vi "Analyze.vi"(11 "Queues":T1) -> ()   [LabVIEW 2014]
uses:
  CMD UI enum.ctl
  CMD Report enum.ctl
  CMD DA enum.ctl
  CMD DAQ enum.ctl
  CMD LOG enum.ctl
  patiant and daq params.ctl
  set-get-size.ctl
  set_get.ctl
  <vilib>/Analysis/baseanly.llb/Mean (DBL).vi
  <vilib>/Analysis/NI_AALBase.lvlib
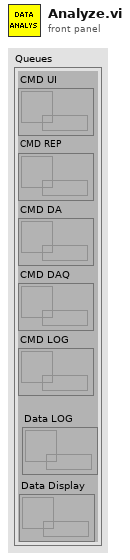
[diagram p1: front panel]
types:
  T1 = cluster{"CMD UI":refnum<queue>, "CMD REP":refnum<queue>, "CMD DA":refnum<queue>, "CMD DAQ":refnum<queue>, "CMD LOG":refnum<queue>, "Data LOG":refnum<queue>, "Data Display":refnum<queue>}
  T2 = typedef "CMD DA enum.ctl" = enum16{"Wait", "Analyze", "Meta Analyze", "Exit"}
  T3 = typedef "patiant and daq params.ctl" = cluster{"DAQ Parameters":cluster{"Sampling rate":dbl, "Max_volt":dbl, "Min_volt":dbl, "DAQmx Physical Channels \nHR,SC":tag, "Resting State":bool, "Analyze every (s)":dbl}, "Patient Info \n(Updates automatically when reading from file)":cluster{"Patient Name":string, "Patient ID":string, "Patient Age":dbl, "Gender":string}, "Raw Data Read Path":path, "Avg HR ":dbl, "Avg SC  ":dbl}
  T4 = typedef "set-get-size.ctl" = enum16{"set", "get", "size"}
  T5 = typedef "set_get.ctl" = enum16{"Set", "Get"}
  T6 = typedef "CMD UI enum.ctl" = enum16{"Init all", "Update Patient Info", "Update Analyzed", "Create Report", "Analyze Data", "Start DAQ", "Start Read", "LOG Data", "Stop LOG Data", "Stop DAQ", "Stop Read", "EXIT"}
  T7 = cluster{bool, bool, bool, "mean":dbl, "mean":dbl}
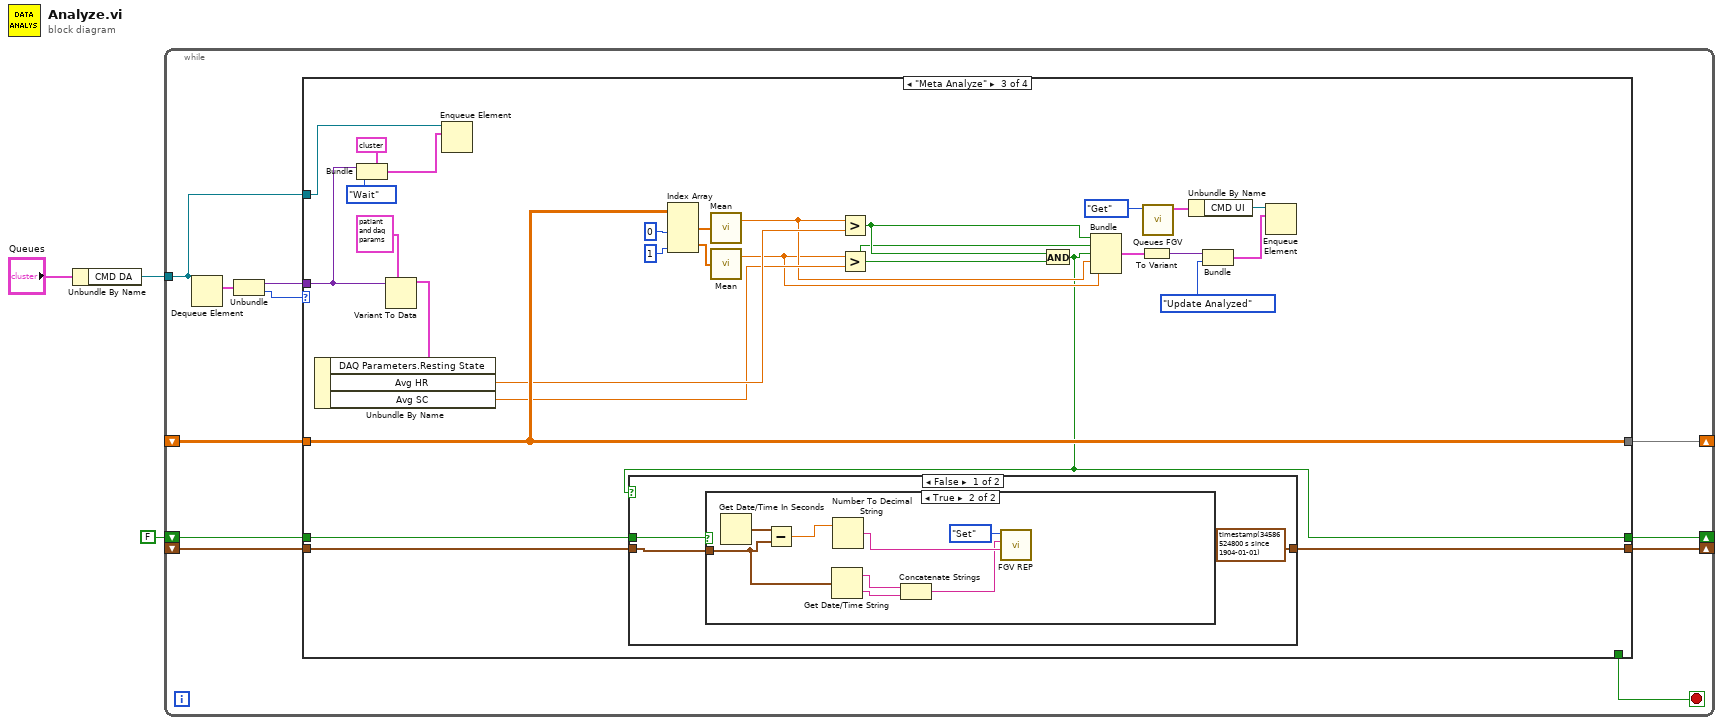
[diagram p0: block diagram]
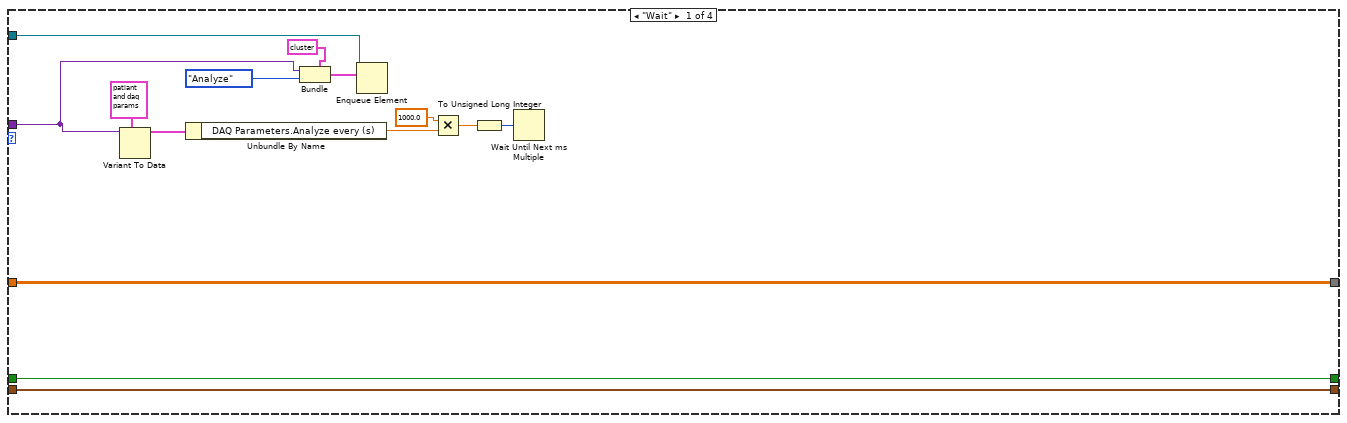
[diagram p2: hidden frame]
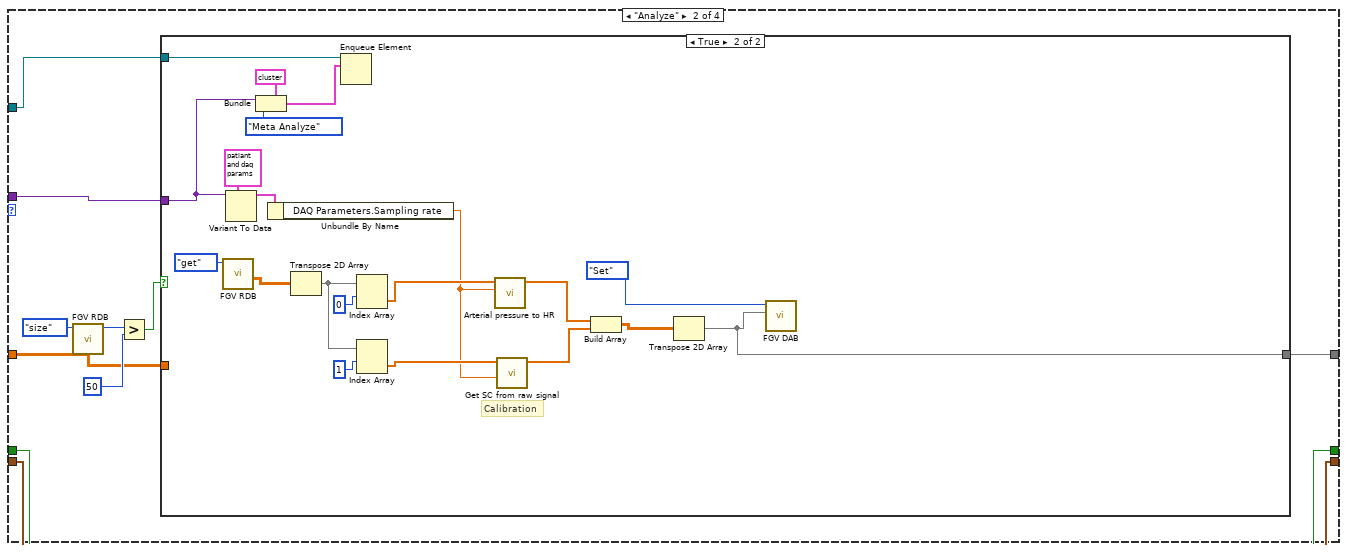
[diagram p3: hidden frame]
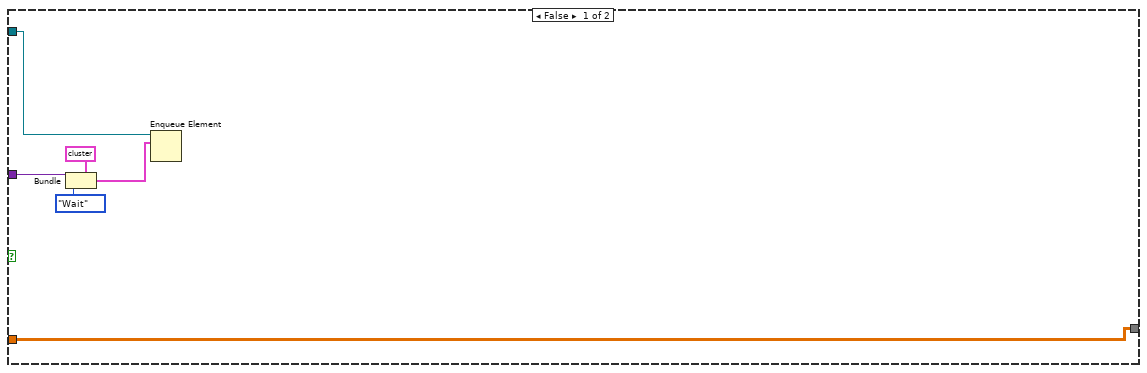
[diagram p4: hidden frame]
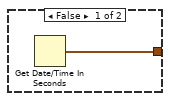
[diagram p7: hidden frame]
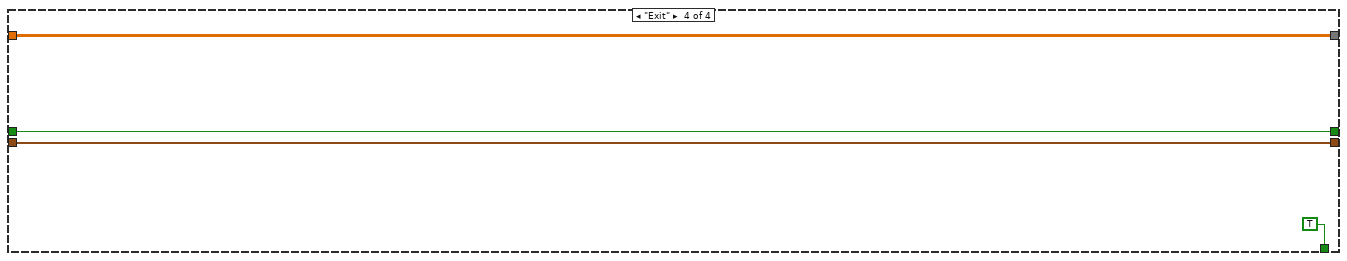
[diagram p8: hidden frame]
diagram:
  n1 = Unbundle By Name("Queues") -> ("CMD DA"=w2:refnum<queue>)
  n2 = while {
    tunnel: w2 -> [w10]
    shift-right: [w8] -> _
    shift-left: _ -> [w9]
    shift-right: [w7] -> _
    shift-left: _ -> [w6]
    shift-right: [w5] -> _
    shift-left: FALSE -> [w4]
    stop <- w12 stop-if-true
    n3 = Dequeue Element(queue=w10) -> (element=w14:cluster{variant, T2})  [unwired: 2 in, 3 out]
    n4 = Unbundle(w14) -> (w11:variant, w13:T2)
    n5 = case shown="\"Meta Analyze\"" w13 {
      tunnel: [_ _ _ TRUE] -> w12
      tunnel: w11 -> [w18 w35 w87 _]
      tunnel: w10 -> [w25 w33 w88 _]
      tunnel: [w17 w32 w86 w112] -> w8
      tunnel: w9 -> [w17 w31 w86 w112]
      tunnel: [w16 w30 w68 w110] -> w7
      tunnel: w6 -> [w16 w30 w67 w110]
      tunnel: [w15 w29 w66 w111] -> w5
      tunnel: w4 -> [w15 w29 w65 w111]
      frame "Wait" {
        n6 = Variant To Data(type=T3 {"DAQ Parameters"={"Sampling rate"=0.0, "Max_volt"=0.0, "Min_volt"=0.0, "DAQmx Physical Channels \nHR,SC"="", "Resting State"=FALSE, "Analyze every (s)"=0.01}, "Patient Info \n(Updates automatically when reading from file)"={"Patient Name"="", "Patient ID"="", "Patient Age"=0.0, "Gender"=""}, "Raw Data Read Path"=path "", "Avg HR "=0.0, "Avg SC  "=0.0} ("output cluster"), Variant=w18) -> (data=w28:T3)  [unwired: 1 in, 1 out]
        n7 = Unbundle By Name(w28) -> ("DAQ Parameters.Analyze every (s)"=w22:dbl)
        n8 = Bundle(cluster=cluster{variant, T2} {variant, enum."Analyze"} ("element"), w18, CMD_DA_enum."Analyze") -> (w19:cluster{variant, T2})
        n9 = Enqueue Element(queue=w25, element=w19) -> ()  [unwired: 2 in, 3 out]
        n10 = Multiply(x=1000.0, y=w22) -> (x*y=w27:dbl)
        n11 = To Unsigned Long Integer(number=w27) -> (unsigned 32bit integer=w24:u32)
        n12 = Wait Until Next ms Multiple(millisecond multiple=w24) -> ()  [unwired: 1 out]
      }
      frame "Analyze" {
        n13 = call "FGV RDB.vi"("Command"=set-get-size."size") -> ("Size"=w37:i32)  [unwired: 9 in, 1 out]
        n14 = Greater?(x=w37, y=50) -> (0:w34:bool)
        n15 = case shown="True" w34 {
          tunnel: w35 -> [w41 w58]
          tunnel: w33 -> [w40 w50]
          tunnel: [w39 w46] -> w32
          tunnel: w31 -> [w39 _]
          frame False {
            n16 = Bundle(cluster=cluster{variant, T2} {variant, enum."Analyze"} ("element"), w41, CMD_DA_enum."Wait") -> (w44:cluster{variant, T2})
            n17 = Enqueue Element(queue=w40, element=w44) -> ()  [unwired: 2 in, 3 out]
          }
          frame True {
            # "Calibration"
            n18 = call "FGV RDB.vi"("Command"=set-get-size."get") -> ("Raw data out"=w56:dbl[][])  [unwired: 9 in, 1 out]
            n19 = Variant To Data(type=T3 {"DAQ Parameters"={"Sampling rate"=0.0, "Max_volt"=0.0, "Min_volt"=0.0, "DAQmx Physical Channels \nHR,SC"="", "Resting State"=FALSE, "Analyze every (s)"=0.01}, "Patient Info \n(Updates automatically when reading from file)"={"Patient Name"="", "Patient ID"="", "Patient Age"=0.0, "Gender"=""}, "Raw Data Read Path"=path "", "Avg HR "=0.0, "Avg SC  "=0.0} ("output cluster"), Variant=w58) -> (data=w64:T3)  [unwired: 1 in, 1 out]
            n20 = Bundle(cluster=cluster{variant, T2} {variant, enum."Analyze"} ("element"), w58, CMD_DA_enum."Meta Analyze") -> (w61:cluster{variant, T2})
            n21 = Unbundle By Name(w64) -> ("DAQ Parameters.Sampling rate"=w45:dbl)
            n22 = Transpose 2D Array(2D array=w56) -> (transposed array=w57:dbl[][])
            n23 = Enqueue Element(queue=w50, element=w61) -> ()  [unwired: 2 in, 3 out]
            n24 = Index Array(array=w57, index (row)=0) -> (element=w54:dbl[])  [unwired: 1 in]
            n25 = Index Array(array=w57, index (row)=1) -> (element=w55:dbl[])  [unwired: 1 in]
            n26 = call "Arterial pressure to HR.vi"("Numeric"=w45, "Raw HR"=w54) -> ("HR"=w48:dbl[])  [unwired: 9 in]
            n27 = call "Get SC from raw signal.vi"("Sampling Rate"=w45, "raw SC"=w55) -> ("SC"=w47:dbl[])  [unwired: 9 in]
            n28 = Build Array(w48, w47) -> (w49:dbl[][])
            n29 = Transpose 2D Array(2D array=w49) -> (transposed array=w46:dbl[][])
            n30 = call "FGV DAB.vi"("HR/SC"=w46, "Enum"=set_get."Set") -> ()  [unwired: 9 in, 1 out]
          }
        }
      }
      frame "Meta Analyze" {
        n31 = Bundle(cluster=cluster{variant, T2} {variant, enum."Analyze"} ("element"), w87, CMD_DA_enum."Wait") -> (w89:cluster{variant, T2})
        n32 = Variant To Data(type=T3 {"DAQ Parameters"={"Sampling rate"=0.0, "Max_volt"=0.0, "Min_volt"=0.0, "DAQmx Physical Channels \nHR,SC"="", "Resting State"=FALSE, "Analyze every (s)"=0.01}, "Patient Info \n(Updates automatically when reading from file)"={"Patient Name"="", "Patient ID"="", "Patient Age"=0.0, "Gender"=""}, "Raw Data Read Path"=path "", "Avg HR "=0.0, "Avg SC  "=0.0} ("output cluster"), Variant=w87) -> (data=w93:T3)  [unwired: 1 in, 1 out]
        n33 = Unbundle By Name(w93) -> ("Avg HR"=w85:dbl, "Avg SC"=w84:dbl)  [unwired: 1 out]
        n34 = Enqueue Element(queue=w88, element=w89) -> ()  [unwired: 2 in, 3 out]
        n35 = Index Array(array=w86, index (col) #1=0 ("disabled index (col)"), index (col) #2=1 ("index (col)")) -> (element #1=w74:dbl[], element #2=w73:dbl[])  [unwired: 2 in]
        n36 = call-poly <vilib>:"Mean.vi"("X"=w74) -> ("mean"=w70:dbl)  [unwired: 1 out]
        n37 = call-poly <vilib>:"Mean.vi"("X"=w73) -> ("mean"=w69:dbl)  [unwired: 1 out]
        n38 = Greater?(x=w70, y=w85) -> (0:w72:bool)
        n39 = Greater?(x=w69, y=w84) -> (0:w71:bool)
        n40 = And(x=w72, y=w71) -> (x .and. y?=w66:bool)
        n41 = case shown="False" w66 {
          tunnel: [timestamp(34586524800 s since 1904-01-01) ("seconds since 1Jan1904") w107] -> w68
          tunnel: w67 -> [w94 w105]
          tunnel: w65 -> [w95 w106]
          frame False {
            n42 = case shown="True" w95 {
              tunnel: w94 -> [_ w103]
              frame False {
              }
              frame True {
                n43 = Get Date/Time In Seconds() -> (seconds since 1Jan1904=w104:timestamp)
                n44 = Subtract(x=w104, y=w103) -> (x-y=w102:dbl)
                n45 = Get Date/Time String(seconds (now)=w103) -> (date string=w99:string, time string=w98:string)  [unwired: 2 in]
                n46 = Number To Decimal String(number=w102) -> (decimal integer string=w100:string)  [unwired: 1 in]
                n47 = Concatenate Strings(w99, w98) -> (w97:string)
                n48 = call "FGV REP.vi"("Period of Excitation"=w100, "Date/Time of Excitation"=w97, "Enum"=set_get."Set") -> ()  [unwired: 8 in, 1 out]
              }
            }
          }
          frame True {
            n49 = case shown="True" w106 {
              tunnel: [w108 w109] -> w107
              tunnel: w105 -> [_ w109]
              frame False {
                n50 = Get Date/Time In Seconds() -> (seconds since 1Jan1904=w108:timestamp)
              }
              frame True {
              }
            }
          }
        }
        n51 = Bundle(w72, w71, w66, "mean"=w70, "mean"=w69) -> (w77:T7)  [unwired: 1 in]
        n52 = To Variant(anything=w77) -> (Variant=w76:variant)
        n53 = call "Queues FGV.vi"("Enum"=set_get."Get") -> ("Queues"=w80:T1)  [unwired: 10 in]
        n54 = Unbundle By Name(w80) -> ("CMD UI"=w79:refnum<queue>)
        n55 = Bundle("Variant"=w76, CMD_UI_enum."Update Analyzed") -> (w78:cluster{"Variant":variant, T6})  [unwired: 1 in]
        n56 = Enqueue Element(queue=w79, element=w78) -> ()  [unwired: 2 in, 3 out]
      }
      frame "Exit" {
      }
    }
  }
